vi "Filter.vi"() -> ()   [LabVIEW 2020, in "Examples.lvlib"]
uses:
  Examples.lvlib
  b8170063-6c36-4763-8043-97c96562bd8c.vi
  Is Even.vi
panel:
  out "Filtered Array":i32[](array[numeric])
  in  "Array":i32[](array[numeric])=[-3, -2, -1, 0, 1, 2, 3, 4, 5]
  # "1) Take note of the numbers in the Array control. Add new ones if you would like.\n2) Run the VI.\n3) Note that the Filter Array contains only the even numbers.\n4) View the block diagram."
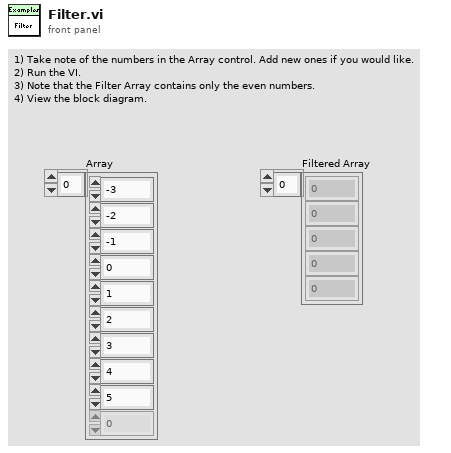
[diagram p1: front panel]
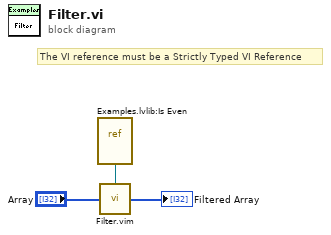
[diagram p0: block diagram]
diagram:
  # "The VI reference must be a Strictly Typed VI Reference"
  n1 = vi-ref "Examples.lvlib:Is Even.vi"() -> (w3:refnum<vi>)
  n2 = call "Filter.vim"("Predicate"=w3, "Array"="Array") -> ("Filtered Array"=→"Filtered Array":i32[])  [unwired: 2 in]
